vi "ESR.vi"(8 "Error In":errorcluster, 11 "VISA resource name":refnum<visa-resource-name>) -> (0 "Error Out":errorcluster, 3 "VISA resource name out":refnum<visa-resource-name>)   [LabVIEW 2013]
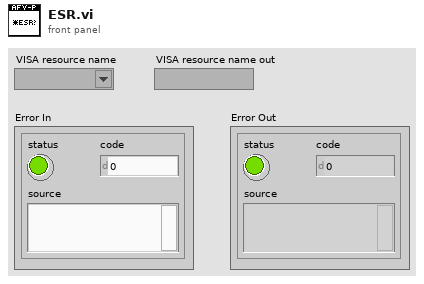
[diagram p1: front panel]
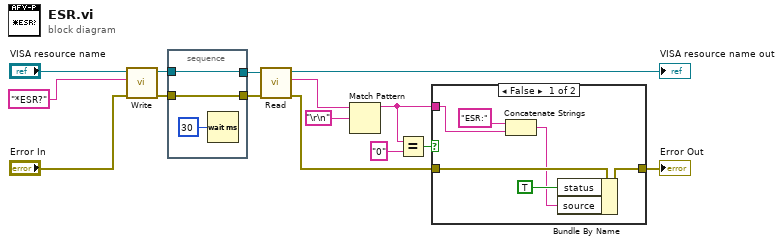
[diagram p0: block diagram]
diagram:
  n1 = call "Write.vi"("Error In"="Error In", "Write Buffer"="*ESR?", "VISA resource name"="VISA resource name") -> ("Error Out"=w6:errorcluster, "VISA resource name out"=w9:refnum<visa-resource-name>)  [unwired: 7 in]
  n2 = stacked-sequence {
    tunnel: [w17] -> w8
    tunnel: w9 -> [w17]
    tunnel: [w16] -> w7
    tunnel: w6 -> [w16]
    frame #0 {
      n3 = Wait (ms)(milliseconds to wait=u32 30) -> ()  [unwired: 1 out]
    }
  }
  n4 = call "Read.vi"("Error In"=w7, "VISA resource name"=w8) -> ("Error Out"=w3:errorcluster, "Read Data"=w14:string, "VISA resource name out"=→"VISA resource name out":refnum<visa-resource-name>)  [unwired: 7 in]
  n5 = Match Pattern(string=w14, regular expression="\r\n") -> (before substring=w1:string)  [unwired: 1 in, 3 out]
  n6 = Equal?(x=w1, y="0") -> (x = y?=w4:bool)
  n7 = case shown="False" w4 {
    tunnel: w3 -> [w24 w25]
    tunnel: [w23 w25] -> w2
    tunnel: w1 -> [w19 _]
    frame False {
      n8 = Concatenate Strings("ESR:", w19) -> (w21:string)
      n9 = Bundle By Name(cluster=w24, "status"=TRUE, "source"=w21) -> (w23:errorcluster)
    }
    frame True {
    }
  }
  "Error Out" <- w2
